vi "TreeList.vi"() -> ()   [LabVIEW 2017]
uses:
  db05dfc8-0df7-4dfa-a115-8713d831efe2.vi
  fa755ba5-a14e-4b93-a51b-607645048859.vi
  0d6320fe-d36d-49c9-9f62-4befc47405e7.vi
  Malleable VIs Basics Lesson 2.vi
panel:
  out "notification":bool
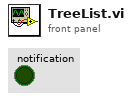
[diagram p1: front panel]
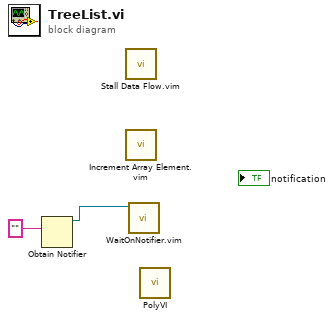
[diagram p0: block diagram]
diagram:
  n1 = Obtain Notifier(notification data type="") -> (notifier out=w1:refnum<notifier>)  [unwired: 3 in, 2 out]
  n2 = call "Stall Data Flow.vim"() -> ()  [unwired: 2 in, 2 out]
  n3 = call "Increment Array Element.vim"() -> ()  [unwired: 2 in, 1 out]
  n4 = call "WaitOnNotifier.vim"("notifier"=w1) -> ()  [unwired: 8 in, 3 out]
  n5 = call-poly "PolyVI.vi"() -> ()  [unwired: 11 in, 1 out]
